vi "Write PWM Length.vi"(8 "error in (no error)":errorcluster, 10 "PWM Length":dbl[unit]=1.0 format="%.1g", 11 "Set Length Msg in":refnum<class "Set Length Msg.lvclass">) -> (0 "error out":errorcluster, 3 "Set Length Msg out":refnum<class "Set Length Msg.lvclass">)   [LabVIEW 2017, in "BNT_DAQmx.lvlib" / "Set Length Msg.lvclass"]
uses:
  Set Length Msg.lvclass
  Set Length Msg.lvclass/Set Length Msg.ctl
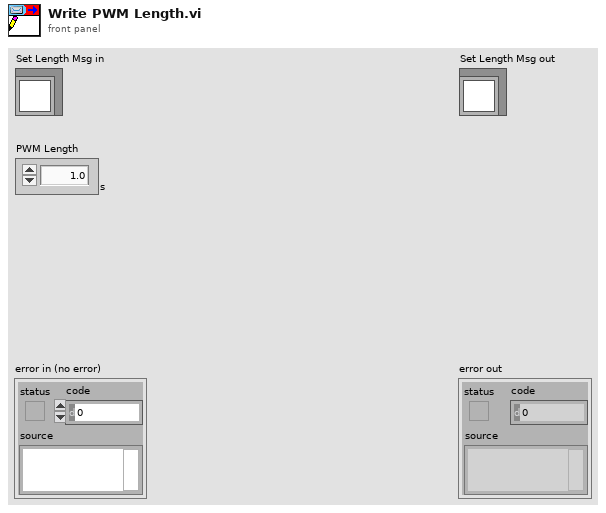
[diagram p1: front panel]
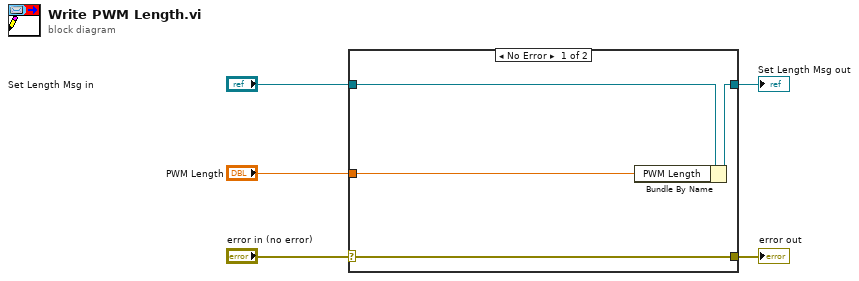
[diagram p0: block diagram]
diagram:
  n1 = case shown="No Error" "error in (no error)" {
    selector: "error in (no error)" -> [w9 w10]
    tunnel: [w9 w10] -> w4
    tunnel: [w7 w11] -> w2
    tunnel: "Set Length Msg in" -> [w8 w11]
    tunnel: "PWM Length" -> [w6 _]
    frame No Error {
      n2 = Bundle By Name(cluster=w8, "PWM Length"=w6) -> (w7:refnum<class "Set Length Msg.lvclass">)
    }
    frame Error {
    }
  }
  "error out" <- w4
  "Set Length Msg out" <- w2
